vi "FakeImageSignalGenerator.vi"(8 "Z":dbl, 9 "Y":dbl=1.0, 10 "X":dbl) -> (2 "E":dbl)   [LabVIEW 2013]
doc: "This template is the starting point for creating a model function to be passed to the Nonlinear Curve Fit.vi."
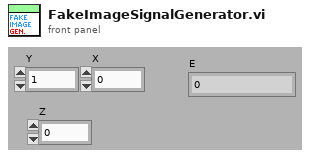
[diagram p1: front panel]
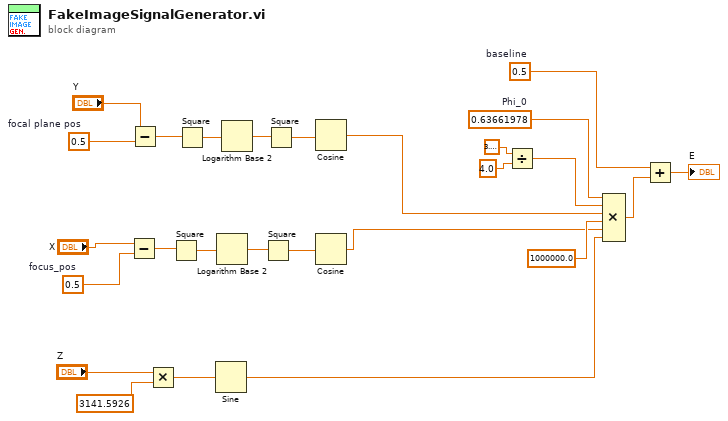
[diagram p0: block diagram]
diagram:
  w18 = 0.5  # focal plane pos
  w15 = 0.5  # focus_pos
  w20 = 0.5  # baseline
  w21 = 0.63661978  # Phi_0
  n1 = Subtract(x="X", y=w15) -> (x-y=w13:dbl)
  n2 = Subtract(x="Y", y=w18) -> (x-y=w14:dbl)
  n3 = Multiply(x="Z", y=3141.5926) -> (x*y=w2:dbl)
  n4 = Square(x=w13) -> (x^2=w11:dbl)
  n5 = Square(x=w14) -> (x^2=w12:dbl)
  n6 = Sine(x=w2) -> (sin(x)=w1:dbl)
  n7 = Logarithm Base 2(1:w11) -> (0:w10:dbl)
  n8 = Logarithm Base 2(1:w12) -> (0:w9:dbl)
  n9 = Square(x=w10) -> (x^2=w7:dbl)
  n10 = Square(x=w9) -> (x^2=w8:dbl)
  n11 = Cosine(x=w8) -> (cos(x)=w6:dbl)
  n12 = Cosine(x=w7) -> (cos(x)=w5:dbl)
  n13 = Divide(x=3.141592653589793, y=4.0) -> (x/y=w24:dbl)
  n14 = Compound Arithmetic op=MULTIPLY(w21, w24, w6, 1000000.0 ("value"), w5, w1) -> (w23:dbl)
  n15 = Add(x=w20, y=w23) -> (x+y=→"E":dbl)
